vi "Save As Measurement Service template.vi"(8 "error in":errorcluster, 10 "Measurement Service Name":string, 11 "Project ref":refnum<vi>) -> (0 "error out":errorcluster)   [LabVIEW 2020, in "MeasurementService Editor.lvlib"]
uses:
  MeasurementService Editor.lvlib
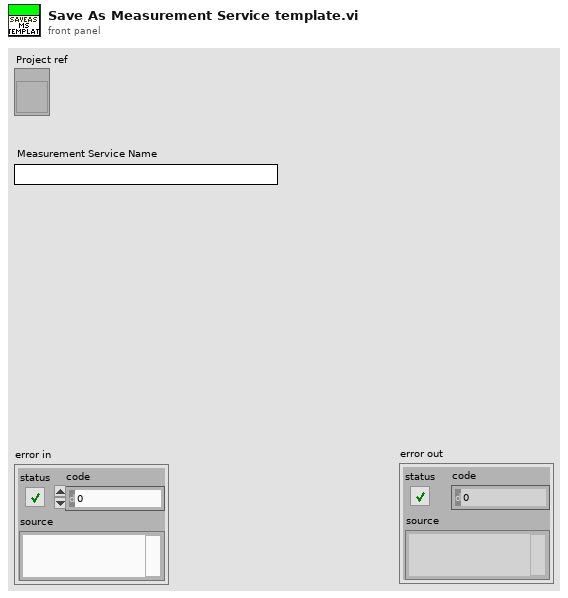
[diagram p1: front panel]
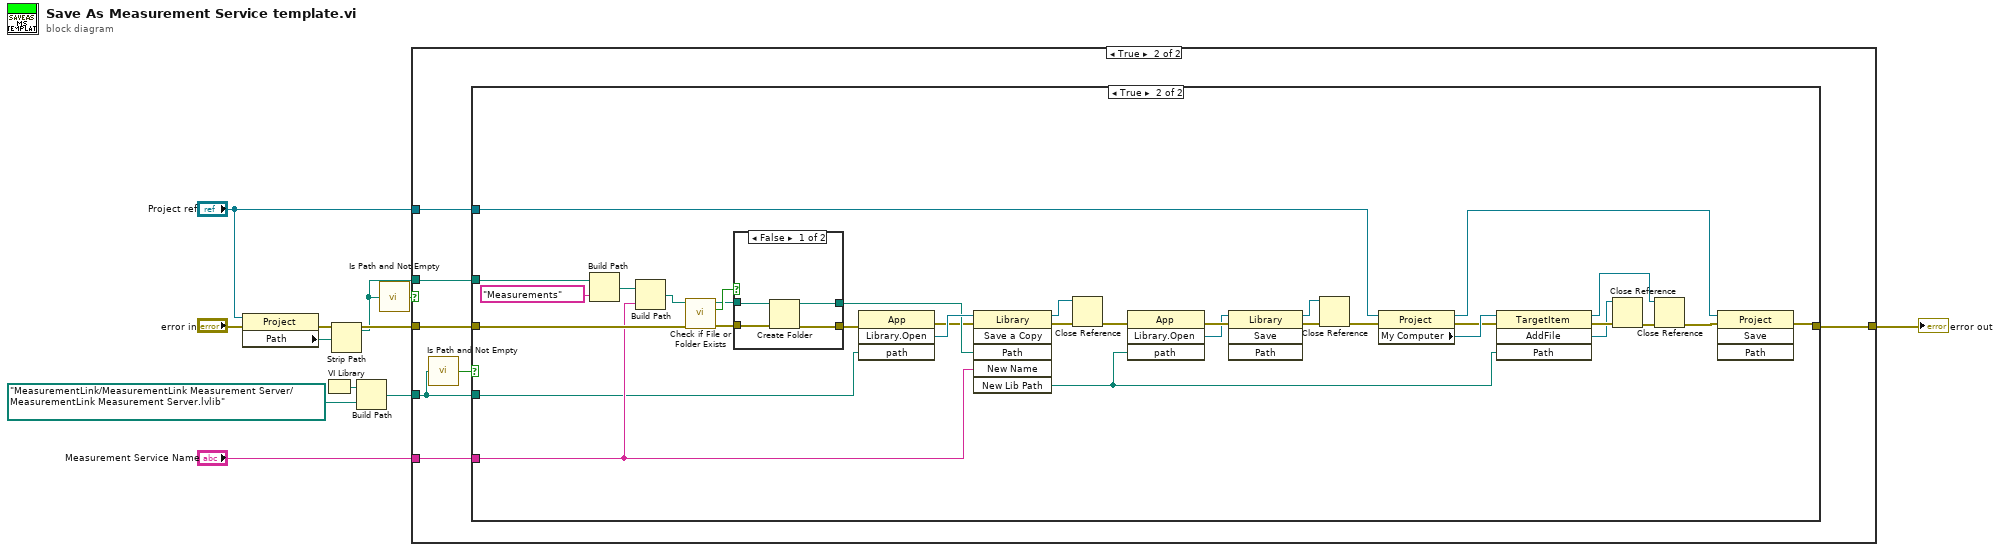
[diagram p0: block diagram]
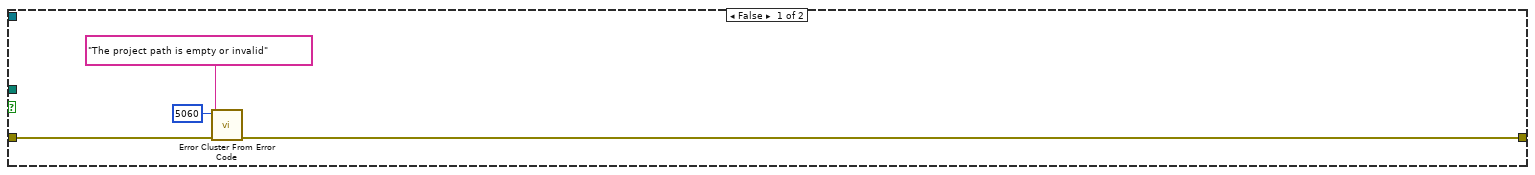
[diagram p2: hidden frame]
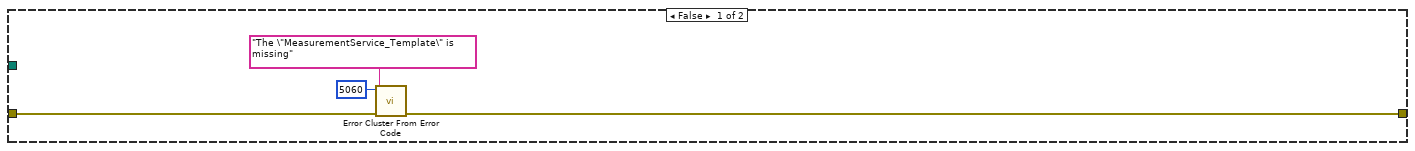
[diagram p3: hidden frame]
diagram:
  n1 = property class="Project"(reference="Project ref", error in="error in") -> (error out=w8:errorcluster, "Path"=w2:path)  [unwired: 1 out]
  n2 = VI Library() -> (path=w7:path)
  n3 = Strip Path(path=w2) -> (stripped path=w1:path)  [unwired: 1 out]
  n4 = Build Path(base path=w7, name or relative path=path "MeasurementLink/MeasurementLink Measurement Server/MeasurementLink Measurement Server.lvlib") -> (appended path=w5:path)
  n5 = call <vilib>:"Is Path and Not Empty.vi"("path"=w1) -> ("Is Path and Not Empty?"=w11:bool)  [unwired: 4 in]
  n6 = case shown="True" w11 {
    tunnel: w8 -> [w15 w22]
    tunnel: [w14 w21] -> w10
    tunnel: w5 -> [_ w19]
    tunnel: "Measurement Service Name" -> [_ w18]
    tunnel: w1 -> [_ w17]
    tunnel: "Project ref" -> [_ w16]
    frame False {
      n7 = call <vilib>:"Error Cluster From Error Code.vi"("error in (no error)"=w15, "error message (\"\")"="The project path is empty or invalid" ("error message (\"\")"), "error code (0)"=5060) -> ("error out"=w14:errorcluster)  [unwired: 6 in]
    }
    frame True {
      n8 = call <vilib>:"Is Path and Not Empty.vi"("path"=w19) -> ("Is Path and Not Empty?"=w20:bool)  [unwired: 4 in]
      n9 = case shown="True" w20 {
        tunnel: w22 -> [w24 w52]
        tunnel: [w23 w31] -> w21
        tunnel: w19 -> [_ w49]
        tunnel: w18 -> [_ w51]
        tunnel: w17 -> [_ w59]
        tunnel: w16 -> [_ w46]
        frame False {
          n10 = call <vilib>:"Error Cluster From Error Code.vi"("error in (no error)"=w24, "error message (\"\")"="The \"MeasurementService_Template\" is missing" ("error message (\"\")"), "error code (0)"=5060) -> ("error out"=w23:errorcluster)  [unwired: 6 in]
        }
        frame True {
          n11 = Build Path(base path=w59, name or relative path="Measurements") -> (appended path=w57:path)
          n12 = Build Path(base path=w57, name or relative path=w51) -> (appended path=w56:path)
          n13 = call <vilib>:"Check if File or Folder Exists.vi"("error in (no error)"=w52, "path"=w56) -> ("error out"=w53:errorcluster, "file or folder exists?"=w55:bool, "dup path"=w54:path)  [unwired: 7 in]
          n14 = case shown="False" w55 {
            tunnel: w54 -> [w62 w65]
            tunnel: w53 -> [w63 w64]
            tunnel: [w61 w64] -> w50
            tunnel: [w60 w65] -> w47
            frame False {
              n15 = Create Folder(path (use dialog)=w62, error in=w63) -> (created path=w60:path, error out=w61:errorcluster)  [unwired: 1 in, 1 out]
            }
            frame True {
            }
          }
          n16 = invoke class="App" method="Library.Open"(error in=w50, "path"=w49) -> (error out=w32:errorcluster, "Open Library"=w48:refnum<vi>)  [unwired: 2 in, 2 out]
          n17 = invoke class="Library" method="Save a Copy"(reference=w48, error in=w32, "Path"=w47, "New Name"=w51) -> (reference out=w41:refnum<vi>, error out=w43:errorcluster, "New Lib Path"=w30:path)  [unwired: 2 in, 3 out]
          n18 = Close Reference(reference=w41, error in (no error)=w43) -> (error out=w42:errorcluster)
          n19 = invoke class="App" method="Library.Open"(error in=w42, "path"=w30) -> (error out=w40:errorcluster, "Open Library"=w39:refnum<vi>)  [unwired: 2 in, 2 out]
          n20 = invoke class="Library" method="Save"(reference=w39, error in=w40) -> (reference out=w37:refnum<vi>, error out=w38:errorcluster)  [unwired: 2 in, 2 out]
          n21 = Close Reference(reference=w37, error in (no error)=w38) -> (error out=w36:errorcluster)
          n22 = property class="Project"(reference=w46, error in=w36) -> (reference out=w33:refnum<vi>, error out=w44:errorcluster, "My Computer"=w45:refnum<vi>)
          n23 = invoke class="TargetItem" method="AddFile"(reference=w45, error in=w44, "Path"=w30) -> (reference out=w27:refnum<vi>, error out=w35:errorcluster, "AddFile"=w34:refnum<vi>)  [unwired: 1 in, 1 out]
          n24 = Close Reference(reference=w34, error in (no error)=w35) -> (error out=w29:errorcluster)
          n25 = Close Reference(reference=w27, error in (no error)=w29) -> (error out=w28:errorcluster)
          n26 = invoke class="Project" method="Save"(reference=w33, error in=w28) -> (error out=w31:errorcluster)  [unwired: 2 in, 3 out]
        }
      }
    }
  }
  "error out" <- w10
